vi "Field Cord Generate Trajectory for Alignment.vi"(0 "Initial Postion":T4={"x setpoint"=-0.39, "y setpoint"=-0.8, "th setpoint"=0.0}, 1 "Final Postion":T4={"x setpoint"=-0.39, "y setpoint"=-0.8, "th setpoint"=0.0}, 2 "Limits":T1={"Velocity (fps)"=10.0, "Accel (fps^2)"=22.0, "Jerk (fps^3)"=4000.0, "StoopidFast (fps)"=10.0} {"StoopidFast (fps)" min=0.0; "Jerk (fps^3)" min=0.0 step=1.0; "Accel (fps^2)" min=0.0; "Velocity (fps)" min=0.0}) -> (3 "Error":T4, 4 "Time & Dist":cluster{"Time (s)":dbl, "Distance (ft)":dbl}, 5 "Updated Waypoints":cluster{"x":dbl, "y":dbl, "th":dbl}[](array[cluster]), 6 "Trajectory Data Out":T3(array[cluster]))   [LabVIEW 2023]
uses:
  bordeaux-pathinator/Bordeaux/Types/Segment Type.ctl
  bordeaux-pathinator/Bordeaux/Types/Limits.ctl
  bordeaux-pathinator/Bordeaux/Types/Angluar Limits.ctl
  bordeaux-pathinator/Bordeaux/Types/Drive Type.ctl
  Framework/Robot Global Data.vi
panel:
  in  "Run visualizer":bool
  out "Velocity Waveform":dbl[](graph)=[7.294446746788231, 7.794446746788231, 8.294446746788232, 8.794446746788232, 9.294446746788232, 9.794446746788232, 9.794446746788232, 9.794446746788232, 9.794446746788232, 9.294446746788232, 8.794446746788232, 8.294446746788232, 7.794446746788232, 7.294446746788232, 6.794446746788232, 6.294446746788232, 5.794446746788232, 5.294446746788232, 4.794446746788232, 4.294446746788232, 3.794446746788232, 3.294446746788232, 2.794446746788232, 2.294446746788232, 1.794446746788232, 1.294446746788232, 0.7944467467882319, 0.2944467467882319, 0.0]
  out "Picture":picture
  in  "Sample Period (s)":dbl=0.02 min=0.001 max=1.0 format="%#_6p"
  out "Past Generation Speed":u32
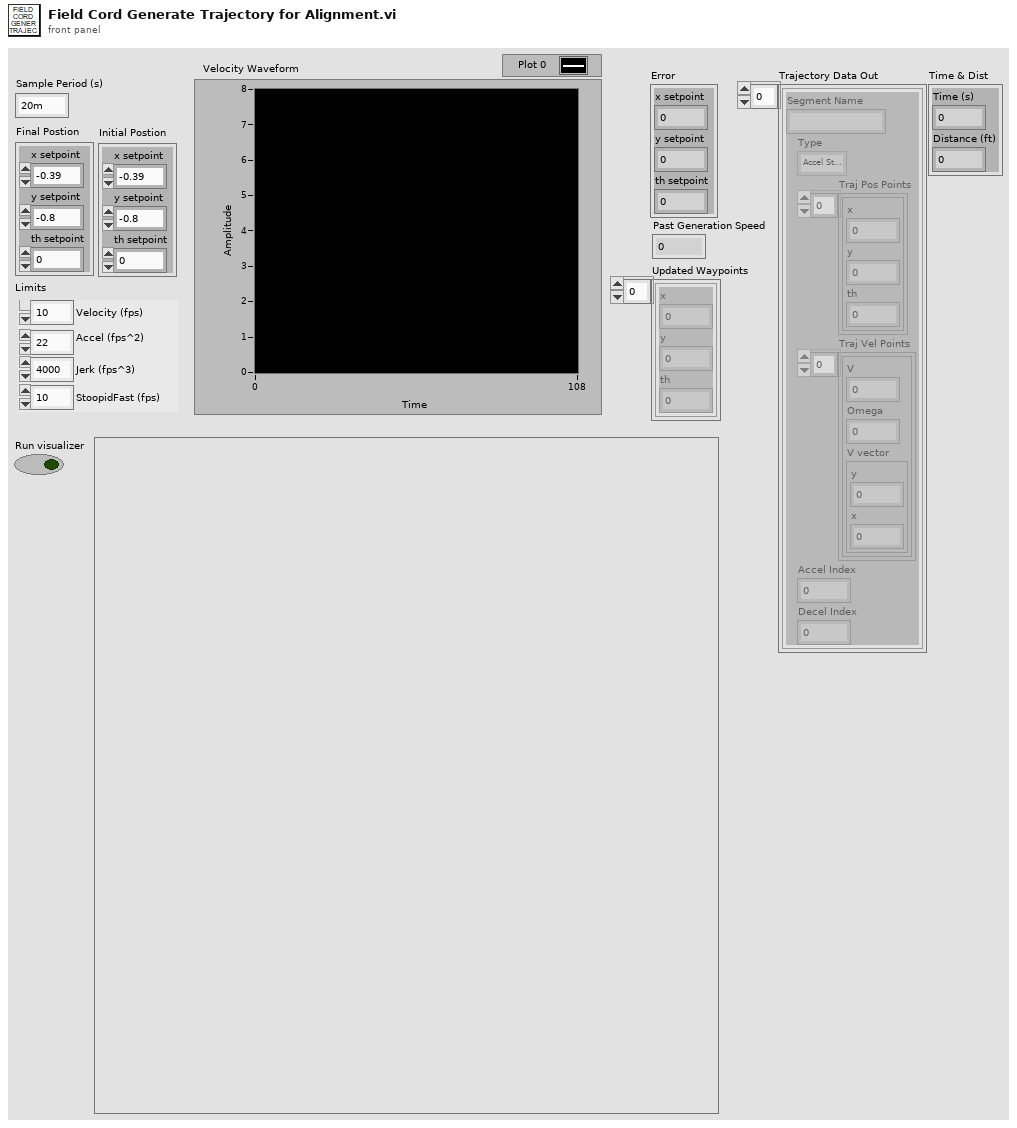
[diagram p1: front panel]
types:
  T1 = typedef "Limits.ctl" = cluster{"Velocity (fps)":dbl, "Accel (fps^2)":dbl, "Jerk (fps^3)":dbl, "StoopidFast (fps)":dbl}
  T2 = typedef "Segment Type.ctl" = enum16{"Accel Straight", "Const Straight", "Blend", "Circle", "Bezier"}
  T3 = cluster{"Segment Name":string, "Type":T2, "Traj Pos Points":cluster{"x":dbl, "y":dbl, "th":dbl}[], "Traj Vel Points":cluster{"V":dbl, "Omega":dbl, "V vector":cluster{"y":dbl, "x":dbl}}[], "Accel Index":i32, "Decel Index":i32}[]
  T4 = cluster{"x setpoint":dbl, "y setpoint":dbl, "th setpoint":dbl}
  T5 = typedef "Drive Type.ctl" = enum16{"Nonholonomic", "Holonomic"}
  T6 = typedef "Angluar Limits.ctl" = cluster{"Velocity (deg/s)":dbl, "Accel (deg/s^2)":dbl, "Jerk (deg/s^3)":dbl}
  T7 = typedef "Robot Velocities.ctl" = cluster{"X Velocity":dbl, "Y Velocity":dbl, "Rotational \nVelocity":dbl}
  T8 = cluster{"x setpoint":dbl, "y setpoint":dbl, "th setpoint":dbl}[]
  T9 = cluster{"V":dbl, "Omega":dbl, "V vector":cluster{"y":dbl, "x":dbl}}[]
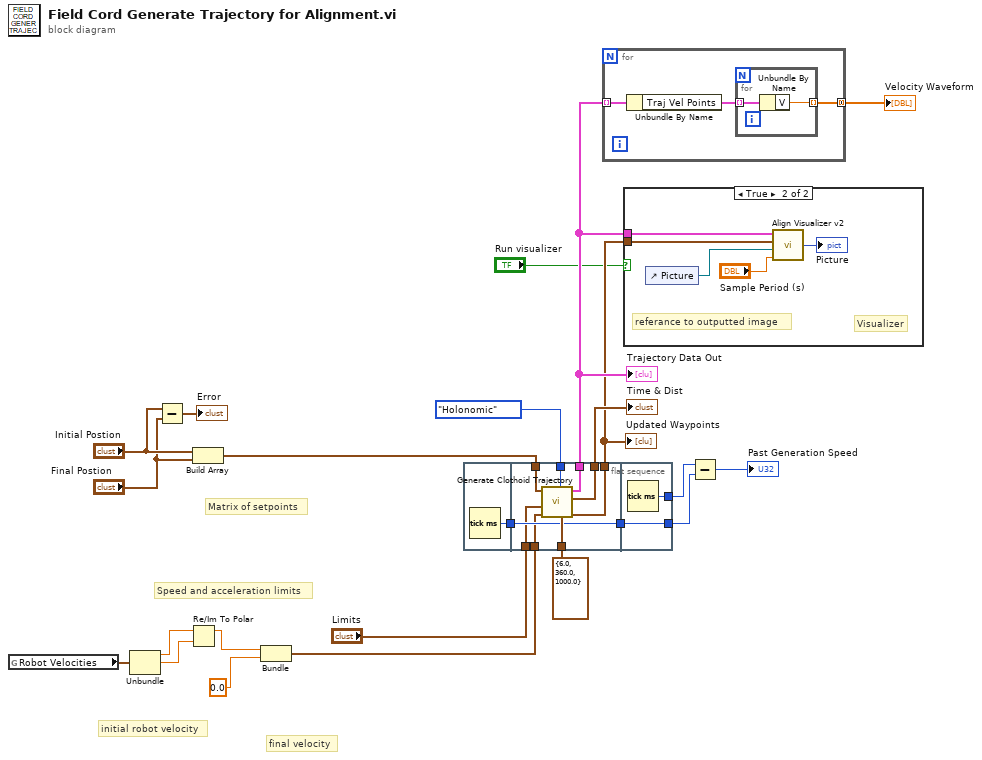
[diagram p0: block diagram]
diagram:
  # "initial robot velocity"
  # "Speed and acceleration limits"
  # "Matrix of setpoints"
  # "final velocity"
  n1 = global read "Robot Global Data.vi" "Robot Velocities"() -> (w23:T7)
  n2 = Unbundle(w23) -> ("X Velocity"=w22:dbl, "Y Velocity"=w21:dbl)  [unwired: 1 out]
  n3 = Subtract(x="Initial Postion", y="Final Postion") -> (x-y=→"Error":T4)
  n4 = Re/Im To Polar(2:w21, 3:w22) -> (1:w13:dbl)  [unwired: 1 out]
  n5 = Build Array("Initial Postion", "Final Postion") -> (w14:T8)
  n6 = Bundle(w13, 0.0) -> (w6:cluster{dbl, dbl})  [unwired: 1 in]
  n7 = flat-sequence {
    tunnel: [w24] -> w20
    tunnel: Drive_Type."Holonomic" ("Drive Type") -> [w33]
    tunnel: T6 {"Velocity (deg/s)"=6.0, "Accel (deg/s^2)"=360.0, "Jerk (deg/s^3)"=1000.0} ("Angular Limits") -> [w32]
    tunnel: [w31] -> w3
    tunnel: w20 -> [w30]
    tunnel: [w30] -> w19
    tunnel: [w29] -> w10
    tunnel: [w28] -> w2
    tunnel: w14 -> [w27]
    tunnel: w6 -> [w26]
    tunnel: "Limits" -> [w25]
    tunnel: [w35] -> w9
    tunnel: w19 -> [w34]
    tunnel: [w34] -> w8
    frame #0 {
      n8 = Tick Count (ms)() -> (millisecond timer value=w24:u32)
    }
    frame #1 {
      n9 = call "Generate Clothoid Trajectory.vi"("Angular Limits"=w32, "Drive Type"=w33, "Conditions"=w26, "Limits"=w25, "WayPoints"=w27) -> ("Updated Waypoints"=w28:cluster{"x":dbl, "y":dbl, "th":dbl}[], "Time & Dist"=w29:cluster{"Time (s)":dbl, "Distance (ft)":dbl}, "Trajectory Data Out"=w31:T3)  [unwired: 3 in, 1 out]
    }
    frame #2 {
      n10 = Tick Count (ms)() -> (millisecond timer value=w35:u32)
    }
  }
  n11 = for {
    tunnel: [w37] -> w4 mode=concatenating
    tunnel: w3 -> [w36] mode=indexing
    n12 = Unbundle By Name(w36) -> ("Traj Vel Points"=w38:T9)
    n13 = for {
      tunnel: w38 -> [w40] mode=indexing
      tunnel: [w39] -> w37 mode=indexing
      n14 = Unbundle By Name(w40) -> ("V"=w39:dbl)
    }
  }
  "Velocity Waveform" <- w4
  n15 = case shown="True" "Run visualizer" {
    tunnel: w3 -> [_ w42]
    tunnel: w2 -> [_ w41]
    frame False {
    }
    frame True {
      # "referance to outputted image"
      # "Visualizer"
      n16 = control-ref of="Picture"() -> (w43:refnum<vi>)
      n17 = call "Align Visualizer v2.vi"("Trajectory Data"=w42, "Points"=w41, "Picture in"=w43, "Sample Period (s)"="Sample Period (s)") -> ("Picture"=→"Picture":picture)  [unwired: 1 in]
    }
  }
  n18 = Subtract(x=w9, y=w8) -> (x-y=→"Past Generation Speed":u32)
  "Trajectory Data Out" <- w3
  "Time & Dist" <- w10
  "Updated Waypoints" <- w2
